vi "determineing some warnings.vi"() -> ()   [LabVIEW 2014]
panel:
  in  "Min Temp 2":dbl
  out "Warning":bool
  out "Warning Tex":string
  in  "Max temp":dbl
  in  "Current Temp":dbl
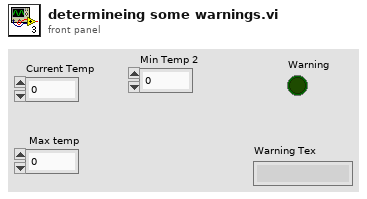
[diagram p1: front panel]
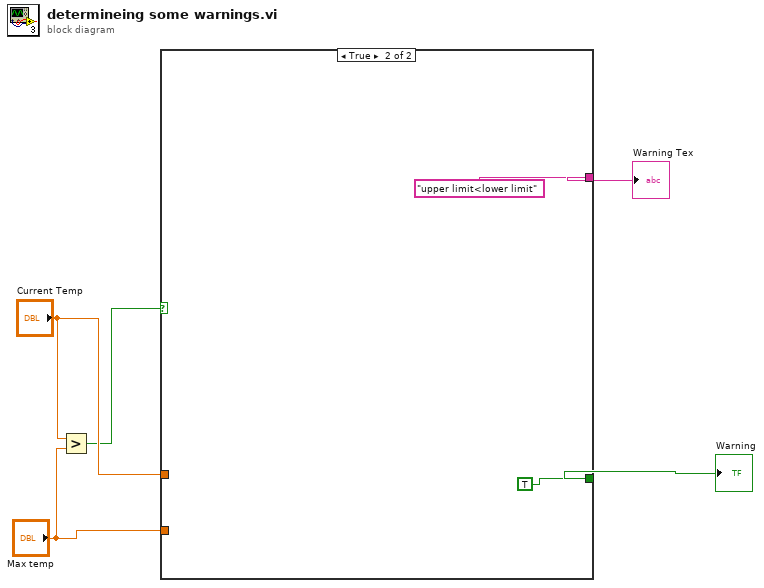
[diagram p0: block diagram]
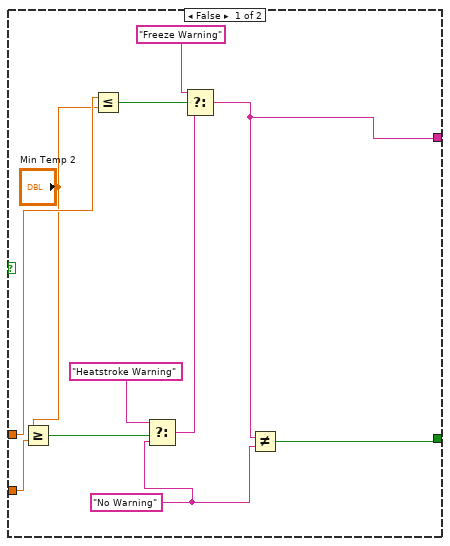
[diagram p2: hidden frame]
diagram:
  n1 = Greater?(x="Current Temp", y="Max temp") -> (0:w1:bool)
  n2 = case shown="True" w1 {
    tunnel: "Current Temp" -> [w7 _]
    tunnel: "Max temp" -> [w8 _]
    tunnel: [w9 TRUE] -> w5
    tunnel: [w10 "upper limit<lower limit"] -> w4
    frame False {
      w14 = "No Warning"
      n3 = Greater Or Equal?(x="Min Temp 2", y=w8) -> (x >= y?=w15:bool)
      n4 = Less Or Equal?(x=w7, y="Min Temp 2") -> (x <= y?=w12:bool)
      n5 = Select(t="Heatstroke Warning", s=w15, f=w14) -> (s? t:f=w13:string)
      n6 = Select(t="Freeze Warning", s=w12, f=w13) -> (s? t:f=w10:string)
      n7 = Not Equal?(x=w10, y=w14) -> (x != y?=w9:bool)
    }
    frame True {
    }
  }
  "Warning Tex" <- w4
  "Warning" <- w5
